vi "Set Current Step.vi"(8 "error in (no error)":errorcluster, 10 "Current Step":u32, 11 "Sequencer in":refnum<class "Sequencer.lvclass">) -> (0 "error out":errorcluster, 3 "Sequencer out":refnum<class "Sequencer.lvclass">)   [LabVIEW 2024, in "Ramses Sequencer.lvlib" / "Sequencer.lvclass"]
uses:
  Sequencer.lvclass
  Program Files (x86)/Enterative/Ramses Framework/Ramses Framework.lvlibp/Service/Service.lvclass
  C:/Program Files (x86)/Enterative/Ramses Framework/Ramses Framework.lvlibp/Service/Service.lvclass
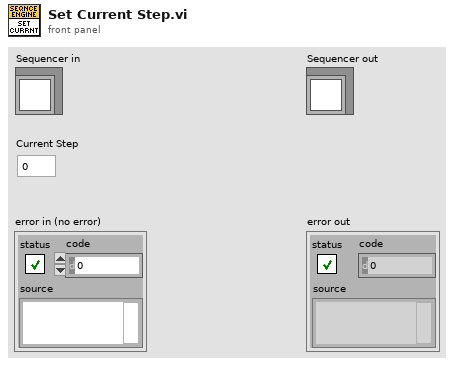
[diagram p1: front panel]
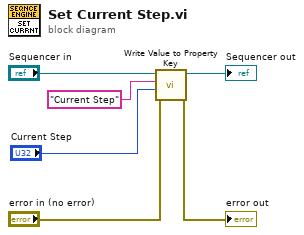
[diagram p0: block diagram]
diagram:
  n1 = call "Write Value to Property Key.vi"("error in (no error)"="error in (no error)", "Value"="Current Step", "Key"="Current Step", "Service in"="Sequencer in") -> ("error out"=→"error out":errorcluster, "Service out"=→"Sequencer out":refnum<class "Sequencer.lvclass">)  [unwired: 6 in]
